vi "Set Center Frequency.vi"(8 "error in (no error)":errorcluster, 10 "Center Frequency (Hz)":u32, 11 "device handle in":T1) -> (0 "error out":errorcluster, 3 "device handle out":T1)   [LabVIEW 2023, in "RTL-SDR.lvlib"]
uses:
  RTL-SDR.lvlib
  Controls/Device Handle.ctl
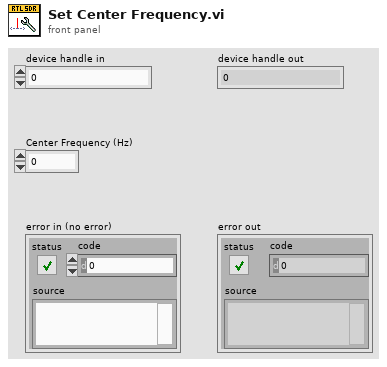
[diagram p1: front panel]
types:
  T1 = typedef "RTL-SDR.lvlib/Device Handle.ctl" = u64
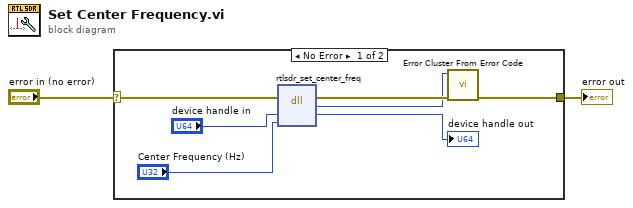
[diagram p0: block diagram]
diagram:
  n1 = case shown="No Error" "error in (no error)" {
    selector: "error in (no error)" -> [w3 w10]
    tunnel: [w5 w10] -> w2
    frame No Error {
      n2 = dll-call lib="usr/local/Cellar/librtlsdr/0.6.0/bin/rtl_sdr" fn="rtlsdr_set_center_freq"(error in=w3, "dev"="device handle in", "freq"="Center Frequency (Hz)") -> (error out=w9:errorcluster, "return type"=w4:i32, "dev"=→"device handle out":u64)  [unwired: 3 in, 1 out]
      n3 = call <vilib>:"Error Cluster From Error Code.vi"("error in (no error)"=w9, "error code (0)"=w4) -> ("error out"=w5:errorcluster)  [unwired: 7 in]
    }
    frame Error {
    }
  }
  "error out" <- w2
